vi "Save Settings To XML File.vi"(2 "error in (no error)":errorcluster, 3 "Save cluster":T1={"Bandwidth"=0, "Coupling"=0, "Current Limit"=0.0, "Current Trip"=0.0, "DMM Address"="", "DMM Measurement Type"=0, "DMM Model"=0, "DMM Reset"=FALSE, "Filter Mode"=0, "Horizontle Scale"=0, "Horizontle Trace Display"=0, "Input Impedance"=0, "Power Supply Address"="", "Power Supply Model"=enum."Keithley 248", "Record Sample Length"=0, "Reset Settings"=FALSE, "ResetPS Settings"=FALSE, "Scope Address"="", "Scope Config on Startup"=0, "Traces to Acquire"=0, "Trigger Coupling"=0, "Trigger Level (V)"=0.0, "Trigger Slope"=0, "Trigger Source"=0, "Trigger Type"=0, "Trip Mode"=0, "Vertical Scale"=0, "Voltage Level"=0.0, "Voltage Limit"=0.0, "Waveform Source"=0, "Scope Model"=1, "DMM Config on Startup"=enum."DMM->PC", "Power Supply Config on Startup"=enum."Power Supply->PC", "Repetitive Signal"=FALSE, "Measurement Mode"=enum."Store All Traces in Single File"} {"Scope Model" items=["Tek TDS 684A/B/C", "Tek TDS 694C", "Tek TDS 744/A", "Tek TDS 754A/C/D", "Tek TDS 784A/C/D"]}, 4 "Settings File Name":string, 5 "Settings File Path":path) -> (0 "error out":errorcluster)   [LabVIEW 2020]
uses:
  <vilib>/Utility/xml.llb/Write to XML File(string).vi
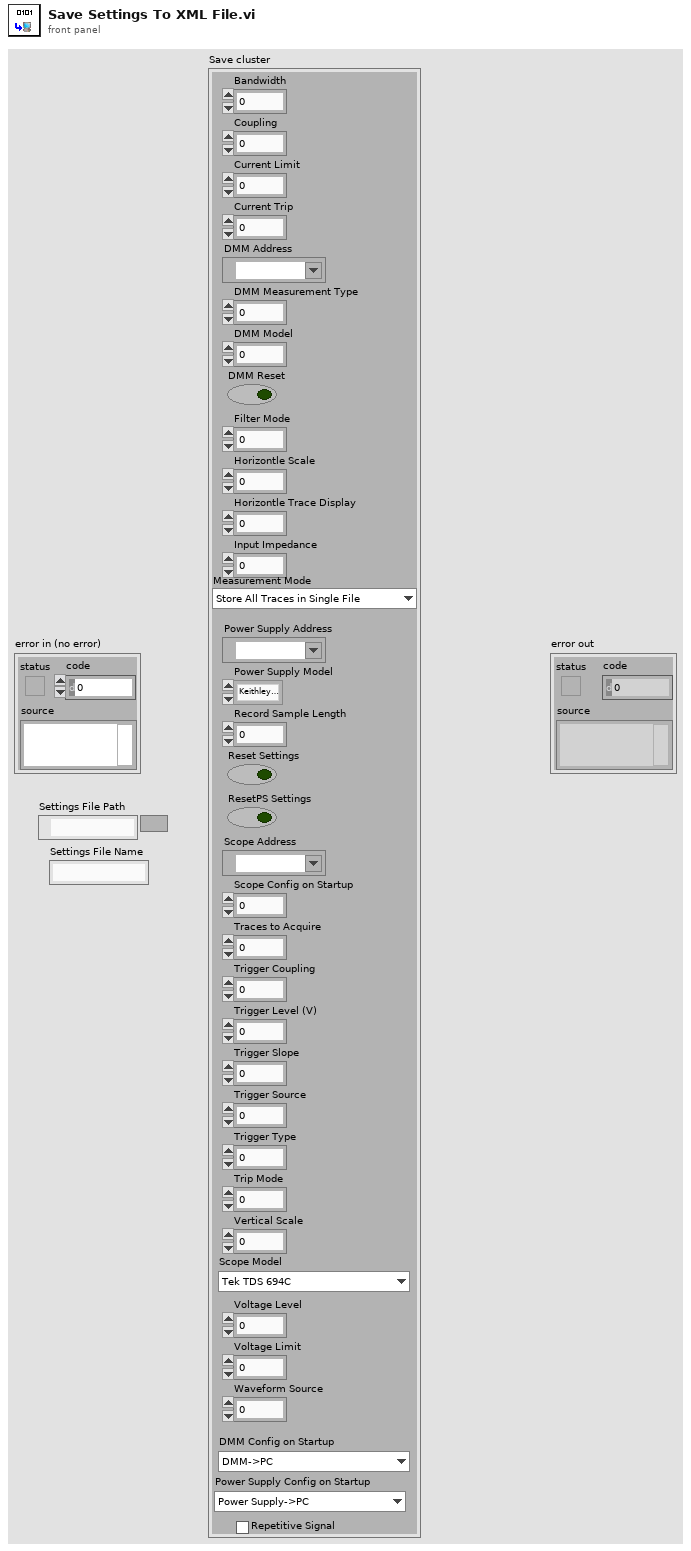
[diagram p1: front panel]
types:
  T1 = cluster{"Bandwidth":u16, "Coupling":u16, "Current Limit":dbl, "Current Trip":dbl, "DMM Address":refnum<visa-resource-name>, "DMM Measurement Type":i32, "DMM Model":u16, "DMM Reset":bool, "Filter Mode":u16, "Horizontle Scale":i32, "Horizontle Trace Display":i32, "Input Impedance":u16, "Power Supply Address":refnum<visa-resource-name>, "Power Supply Model":enum16{"Keithley 248", "Keithley 237", "Keithley 24XX"}, "Record Sample Length":i32, "Reset Settings":bool, "ResetPS Settings":bool, "Scope Address":refnum<visa-resource-name>, "Scope Config on Startup":u16, "Traces to Acquire":u64, "Trigger Coupling":i32, "Trigger Level (V)":dbl, "Trigger Slope":i32, "Trigger Source":u16, "Trigger Type":u16, "Trip Mode":u16, "Vertical Scale":u16, "Voltage Level":sgl, "Voltage Limit":dbl, "Waveform Source":u16, "Scope Model":u16, "DMM Config on Startup":enum16{"PC->DMM", "DMM->PC"}, "Power Supply Config on Startup":enum16{"PC->Power Supply", "Power Supply->PC"}, "Repetitive Signal":bool, "Measurement Mode":enum16{"Store All Traces in Single File", "Store Average/Std. Dev. for each Point", "Store All Traces in Separate Files"}}
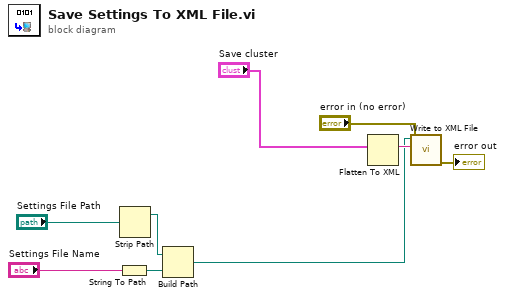
[diagram p0: block diagram]
diagram:
  n1 = String To Path(string="Settings File Name") -> (path=w6:path)
  n2 = Strip Path(path="Settings File Path") -> (stripped path=w7:path)  [unwired: 1 out]
  n3 = Build Path(base path=w7, name or relative path=w6) -> (appended path=w3:path)
  n4 = Flatten To XML(6:"Save cluster") -> (2:w9:string)
  n5 = call-poly <vilib>:"Write to XML File.vi"("error in (no error)"="error in (no error)", "XML Input"=w9, "XML File Path"=w3) -> ("error out"=→"error out":errorcluster)  [unwired: 6 in, 2 out]
